vi "Read TC.vi"(8 "error in (no error)":errorcluster, 11 "TC in":T1) -> (0 "error out":errorcluster, 3 "TC out":T1)   [LabVIEW 2021]
uses:
  <instrlib>/Lake Shore 350/Public/Data/Sensor Data (Single Reading).vi
  <instrlib>/Lake Shore 350/Lake Shore 350.lvlib
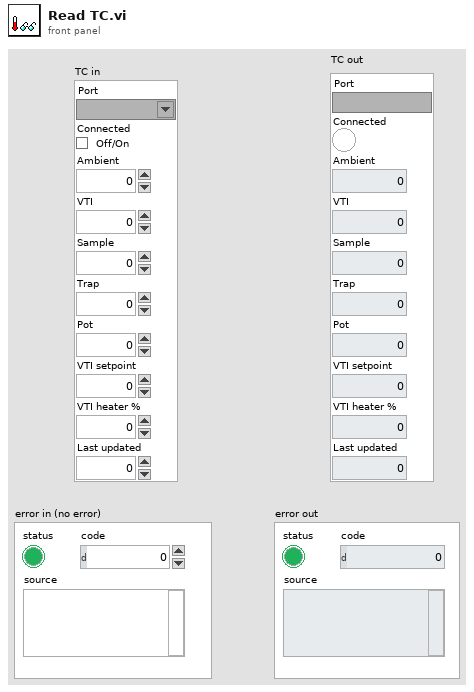
[diagram p1: front panel]
types:
  T1 = cluster{"Port":refnum<visa-resource-name>, "Connected":bool, "Ambient":dbl, "VTI":dbl, "Sample":dbl, "Trap":dbl, "Pot":dbl, "VTI setpoint":dbl, "VTI heater %":dbl, "Last updated":dbl}
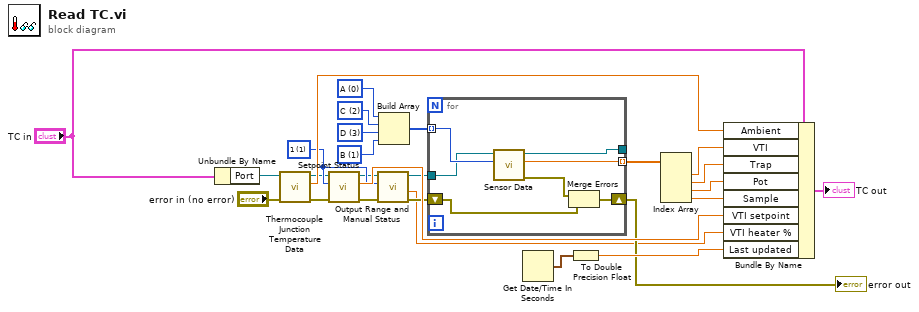
[diagram p0: block diagram]
diagram:
  w7 = u16 1 items=["A", "B", "C", "D", "D2", "D3", "D4", "D5"] ("Input (0:A)")
  w6 = u16 3 items=["A", "B", "C", "D", "D2", "D3", "D4", "D5"] ("Input (0:A)")
  w5 = u16 2 items=["A", "B", "C", "D", "D2", "D3", "D4", "D5"] ("Input (0:A)")
  w12 = u16 1 items=["1"=1, "2"=2] ("Heater Output (1:1)")
  w3 = u16 0 items=["A", "B", "C", "D", "D2", "D3", "D4", "D5"] ("Input (0:A)")
  n1 = Unbundle By Name("TC in") -> ("Port"=w9:refnum<visa-resource-name>)
  n2 = call <instrlib>:"Thermocouple Junction Temperature Data.vi"("error in (no error)"="error in (no error)", "VISA resource name"=w9) -> ("error out"=w17:errorcluster, "Room-Temperature Sensor Data"=w13:dbl, "VISA resource name out"=w8:refnum<visa-resource-name>)  [unwired: 7 in]
  n3 = call <instrlib>:"Setpoint Status.vi"("error in (no error)"=w17, "Output (1:1)"=w12, "VISA resource name"=w8) -> ("error out"=w18:errorcluster, "Setpoint"=w27:dbl, "VISA resource name out"=w11:refnum<visa-resource-name>)  [unwired: 6 in]
  n4 = call <instrlib>:"Output Range and Manual Status.vi"("error in (no error)"=w18, "Output (1:1)"=w12, "VISA resource name"=w11) -> ("error out"=w19:errorcluster, "Manual Output (0.00 %)"=w10:dbl, "VISA resource name out"=w14:refnum<visa-resource-name>)  [unwired: 5 in, 1 out]
  n5 = Build Array(w3, w5, w6, w7) -> (w4:u16[])
  n6 = for {
    tunnel: w4 -> [w34] mode=indexing
    tunnel: [w33] -> w20 mode=indexing
    tunnel: [w32] -> _
    shift-right: [w30] -> w15
    shift-left: w19 -> [w29]
    tunnel: w14 -> [w28]
    n7 = call-poly <instrlib>:"Sensor Data.vi"("Input (0:A)"=w34, "VISA resource name"=w28) -> ("error out"=w31:errorcluster, "Sensor Data"=w33:dbl, "VISA resource name out"=w32:refnum<visa-resource-name>)  [unwired: 7 in]
    n8 = Merge Errors(w31, w29) -> (w30:errorcluster)
  }
  "error out" <- w15
  n9 = Get Date/Time In Seconds() -> (seconds since 1Jan1904=w25:timestamp)
  n10 = To Double Precision Float(number=w25) -> (double precision float=w26:dbl)
  n11 = Index Array(array=w20) -> (element #1=w21:dbl, element #2=w22:dbl, element #3=w23:dbl, element #4=w24:dbl)  [unwired: 4 in]
  n12 = Bundle By Name(cluster="TC in", "Ambient"=w13, "VTI"=w21, "Trap"=w22, "Pot"=w23, "Sample"=w24, "VTI setpoint"=w27, "VTI heater %"=w10, "Last updated"=w26) -> (→"TC out":T1)
